vi "F2V Lin.vi"(11 "ForceArray In":fxp<+/-,25,5>[](array[numeric])=[0.0, 0.0, 0.0, 0.0, 0.0]) -> (3 "ElectrodeVoltageArray Out":fxp<+/-,20,5>[](array[numeric]))   [LabVIEW 2020, in "CtrlEff.lvlib" / "Force2Volt.lvlib"]
doc: "Convert actuation forces into electrode voltages with the appropriate sign.\nFeedback Linearization version: Convert forces into voltages based on the current Z distance."
uses:
  <vilib>/Platform/TimedLoop/XDataNode/timing_clust.ctl
  <vilib>/Platform/TimedLoop/XDataNode/nitl_modes.ctl
  <vilib>/Platform/TimedLoop/XDataNode/wakeup.ctl
  <vilib>/rvi/Emulation/niFpgaSctlEmulationGetInTimedLoop.vi
  <vilib>/rvi/Emulation/niFpgaEmulationReportErrorSimple.vi
  <vilib>/rvi/Emulation/niFpgaGetClockAttributes.vi
  <vilib>/rvi/Emulation/niFpgaCriticalErrorInLSC.vi
  <vilib>/Platform/TimedLoop/XDataNode/XDataNode.xnode
  Force2Volt.lvlib
  <vilib>/Platform/TimedLoop/XDataNode/XDNodeRunTimeDep.lvlib
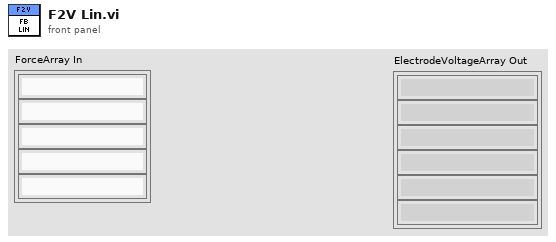
[diagram p1: front panel]
types:
  T1 = typedef "XDNodeRunTimeDep.lvlib/timing_clust.ctl" = cluster{"Expected End [f-1]":u64, "Actual End [f-1]":u64, "Finished Late? [f-1]":bool, "Expected End [i-1]":u64, "Actual End [i-1]":u64, "Finished Late? [i-1]":bool, "Expected Start [i]":u64, "Actual Start [i]":u64, "Expected Start [f]":u64, "Actual Start [f]":u64, "Source Name":string, "Structure Name":string, "Period":i64, "Deadline":i64, "Offset":i64, "Start":i64, "Priority":i32, "Timeout":i32, "Mode":T2, "Wakeup Reason":T3, "Error":errorcluster, "Source Type":string, "Secondary Source Type":string, "Global End Time":u64, "Global Start Time":u64, "Frame Duration":u64, "Iteration Duration":u64, "Assigned CPU":i32, "I/O Scan Engine Mode":u32}
  T2 = typedef "XDNodeRunTimeDep.lvlib/nitl_modes.ctl" = enum32{"No Change", "Process missed periods, maintain original phase", "Discard missed periods, maintain original phase", "Process missed periods, ignore original phase", "Discard missed periods, ignore original phase"}
  T3 = typedef "XDNodeRunTimeDep.lvlib/wakeup.ctl" = enum32{"Normal", "Aborted", "Asynchronous wakeup", "Timing source error", "Timed loop error", "Timeout"}
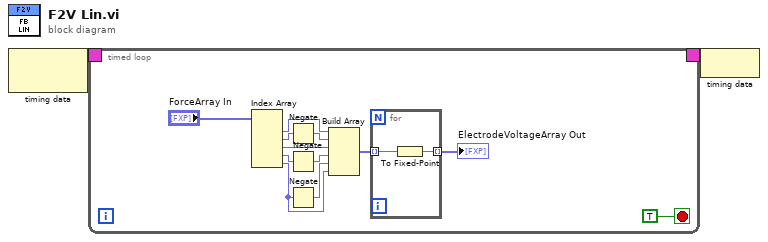
[diagram p0: block diagram]
diagram:
  n1 = node-c288() -> (w2:T1)  [unwired: 1 in]
  n2 = timed-loop {
    timing: w2 -> [_]
    timing-out: [_] -> w1
    stop <- TRUE stop-if-true
    n3 = Index Array(array="ForceArray In") -> (element #1=w13:fxp<+/-,25,5>, element #2=w12:fxp<+/-,25,5>, element #3=w10:fxp<+/-,25,5>, element #4=w9:fxp<+/-,25,5>, element #5=w6:fxp<+/-,25,5>)  [unwired: 5 in]
    n4 = Negate(x=w12) -> (-x=w11:fxp<+/-,26,6>)
    n5 = Negate(x=w9) -> (-x=w8:fxp<+/-,26,6>)
    n6 = Negate(x=w6) -> (-x=w7:fxp<+/-,26,6>)
    n7 = Build Array(w13, w11, w10, w8, w7, w6) -> (w5:fxp<+/-,26,6>[])
    n8 = for {
      tunnel: w5 -> [w16] mode=indexing
      tunnel: [w15] -> w4 mode=indexing
      n9 = To Fixed-Point(number=w16) -> (fixed-point=w15:fxp<+/-,20,5>)  [unwired: 1 in]
    }
    "ElectrodeVoltageArray Out" <- w4
  }
  n10 = node-c288(w1) -> ()
